vi "New Paragraph From Document.vi"(7 "xwpfParagraph Type":refnum<class "xwpfParagraph.lvclass">, 8 "error in (no error)":errorcluster, 11 "Paragraph Ref":refnum<k24>) -> (0 "error out":errorcluster, 2 "New Element Found":bool, 3 "xwpfParagraph out":refnum<class "xwpfParagraph.lvclass">)   [LabVIEW 2017, in "Word_Specific.lvlib" / "xwpfParagraph.lvclass"]
uses:
  xwpfParagraph.lvclass
  C:/Users/Neo/Desktop/Dev_Tools_BR/LabVIEW_NPOI/src/lib/NPOI 2.1.1/NPOI.OOXML.dll
  lib/NPOI 2.1.1/NPOI.OOXML.dll
  xwpfParagraph.lvclass/xwpfParagraph.ctl
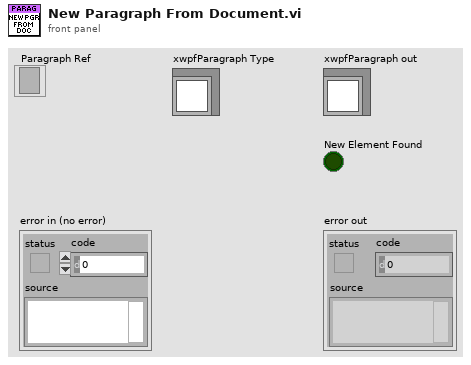
[diagram p1: front panel]
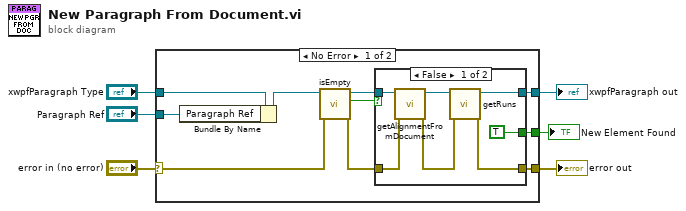
[diagram p0: block diagram]
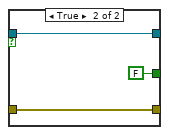
[diagram p2: hidden frame]
diagram:
  n1 = case shown="No Error" "error in (no error)" {
    selector: "error in (no error)" -> [w9 w28]
    tunnel: [w15 w28] -> w5
    tunnel: [w16 w27] -> w3
    tunnel: "xwpfParagraph Type" -> [w14 w27]
    tunnel: "Paragraph Ref" -> [w12 _]
    tunnel: [w7 _] -> w1
    frame No Error {
      n2 = Bundle By Name(cluster=w14, "Paragraph Ref"=w12) -> (w13:refnum<class "xwpfParagraph.lvclass">)
      n3 = call-dynamic "isEmpty.vi"("error in (no error)"=w9, "xwpfParagraph in"=w13) -> ("error out"=w8:errorcluster, "IsEmpty"=w10:bool, "xwpfParagraph out"=w11:refnum<class "xwpfParagraph.lvclass">)  [unwired: 7 in]
      n4 = case shown="False" w10 {
        tunnel: [w21 w26] -> w16
        tunnel: [w20 w25] -> w15
        tunnel: w8 -> [w19 w25]
        tunnel: w11 -> [w18 w26]
        tunnel: [TRUE FALSE] -> w7
        frame False {
          n5 = call "getAlignmentFromDocument.vi"("error in (no error)"=w19, "xwpfParagraph in"=w18) -> ("error out"=w22:errorcluster, "xwpfParagraph out"=w23:refnum<class "xwpfParagraph.lvclass">)  [unwired: 8 in]
          n6 = call "getRuns.vi"("error in (no error)"=w22, "xwpfParagraph in"=w23) -> ("error out"=w20:errorcluster, "xwpfParagraph out"=w21:refnum<class "xwpfParagraph.lvclass">)  [unwired: 8 in]
        }
        frame True {
        }
      }
    }
    frame Error {
    }
  }
  "error out" <- w5
  "xwpfParagraph out" <- w3
  "New Element Found" <- w1
